vi "Write T2_cell.vi"(8 "error in (no error)":errorcluster, 10 "T2":sgl, 11 "cPAS Cell in":refnum<class "cPAS Cell Data.lvclass">) -> (0 "error out":errorcluster, 3 "cPAS Cell out":refnum<class "cPAS Cell Data.lvclass">)   [LabVIEW 2015, in "cPAS Cell Data.lvclass"]
uses:
  cPAS Cell Data/cPAS Cell Data.lvclass
  cPAS Cell Data/cPAS Cell Data.lvclass/cPAS Cell Data.ctl
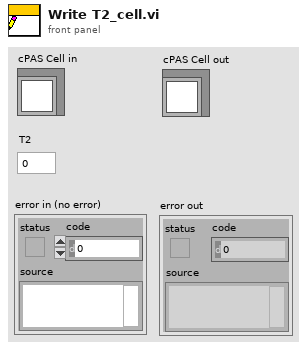
[diagram p1: front panel]
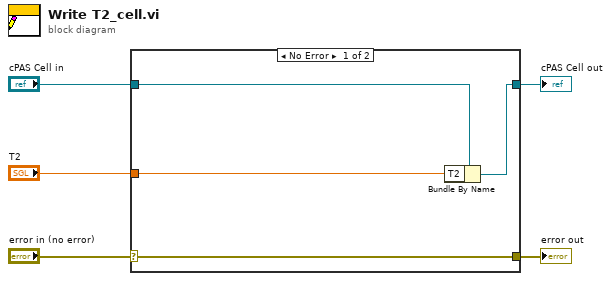
[diagram p0: block diagram]
diagram:
  n1 = case shown="No Error" "error in (no error)" {
    selector: "error in (no error)" -> [w9 w10]
    tunnel: [w9 w10] -> w4
    tunnel: [w7 w11] -> w2
    tunnel: "cPAS Cell in" -> [w8 w11]
    tunnel: "T2" -> [w6 _]
    frame No Error {
      n2 = Bundle By Name(cluster=w8, "T2"=w6) -> (w7:refnum<class "cPAS Cell Data.lvclass">)
    }
    frame Error {
    }
  }
  "error out" <- w4
  "cPAS Cell out" <- w2
